vi "Creator Alias.vi"(11 "jettl Actor in":refnum<class "jettl Actor.lvclass">) -> (2 "Creator Alias":string)   [LabVIEW 2021, in "jettl.lvlib" / "Temporary Actor.lvlib" / "jettl Actor.lvclass"]
uses:
  jettl Actor.lvclass
  jettl Actor.lvclass/jettl Actor.ctl
  Addresses Strategy/Addresses Strategy/Addresses Strategy.lvclass
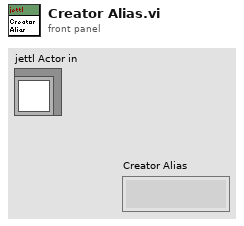
[diagram p1: front panel]
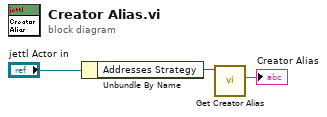
[diagram p0: block diagram]
diagram:
  n1 = Unbundle By Name("jettl Actor in") -> ("Addresses Strategy"=w3:refnum<class "Addresses Strategy.lvclass">)
  n2 = call-dynamic "Get Creator Alias.vi"("Addresses Strategy in"=w3) -> ("Creator Alias"=→"Creator Alias":string)  [unwired: 10 in]
